vi "InStuckInIronsMode.vi"(11 "RelativeWind (0-180)":dbl) -> (3 "InStuckInIronsMode?":bool)   [LabVIEW 2012]
doc: "Checks if the boat is 1) in irons and 2) is going very slowly. There are two cutoffs - an inner angle which has lower standards for what counts as 'in irons' and a broader angle with higher standards for what counts as 'in irons'. This way if the boat is going slowly but is around, say, 25 degrees off the wind, that won't count as stuck. That same speed at 8 degrees off the wind would count as stuck.\n\nIf the boat momentum is low and the boat is in irons range this algorithm should return TRUE and we should use the sails/rudder to coax ourselves out of irons.\n\nEric Schneider, Jan. 2014"
panel:
  in  "Time Until Considered\nStuck In Irons (s)":dbl
  in  "InIronsCutoff (degrees)":dbl=45.0
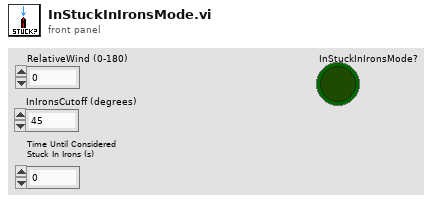
[diagram p1: front panel]
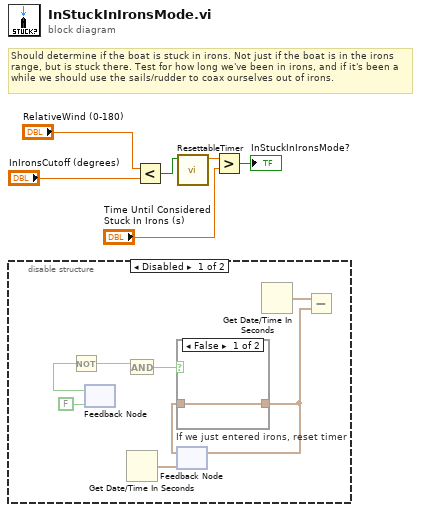
[diagram p0: block diagram]
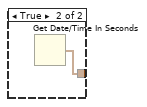
[diagram p2: hidden frame]
diagram:
  # "Should determine if the boat is stuck in irons. Not just if the boat is in the irons range, but is stuck there. Test for how long we've been in irons, and if it's been a while we should use the sails/rudder to coax ourselves out of irons."
  n1 = disable-structure shown="Disabled" {
    frame Disabled {
      n2 = feedback #1(FALSE ("InIrons?")) -> (w12:bool)
      n3 = Not(x=w12) -> (.not. x?=w14:bool)
      n4 = feedback-in #1() -> ()  [unwired: 1 out]
      n5 = And(x=w14) -> (x .and. y?=w11:bool)  [unwired: 1 in]
      n6 = Get Date/Time In Seconds() -> (seconds since 1Jan1904=w9:timestamp)
      n7 = feedback #2(w9) -> (w10:timestamp)
      n8 = case "If we just entered irons, reset timer" shown="False" w11 {
        tunnel: [w15 w16] -> w8
        tunnel: w10 -> [w15 _]
        frame False {
        }
        frame True {
          n9 = Get Date/Time In Seconds() -> (seconds since 1Jan1904=w16:timestamp)
        }
      }
      n10 = feedback-in #2(w8) -> ()
      n11 = Get Date/Time In Seconds() -> (seconds since 1Jan1904=w7:timestamp)
      n12 = Subtract(x=w7, y=w8) -> ()  [unwired: 1 out]
    }
    frame Enabled {
    }
  }
  n13 = Less?(x="RelativeWind (0-180)", y="InIronsCutoff (degrees)") -> (x < y?=w2:bool)
  n14 = call "ResettableTimer.vi"("Restart timer?"=w2) -> ("Time since last reset"=w1:dbl)  [unwired: 10 in]
  n15 = Greater?(x=w1, y="Time Until Considered\nStuck In Irons (s)") -> (0:→"InStuckInIronsMode?":bool)
